vi "Check for DAQ Device.vi"(11 "Physical Channel":tag="Dev1/ai0") -> (0 "error out":errorcluster, 3 "Found?":bool)   [LabVIEW 2011]
doc: "Checks for the specified DAQ device.\n\n\nVersion 1.0 - 02/13/2013\n\nPhaeron, Inc.\nwww.phaeron.com\ninfo@phaeron.com"
uses:
  <vilib>/DAQmx/create/channels.llb/DAQmx Create Channel (AI-Voltage-Basic).vi
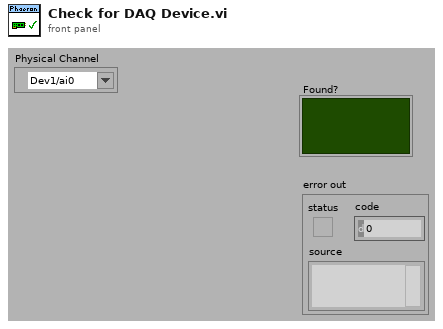
[diagram p1: front panel]
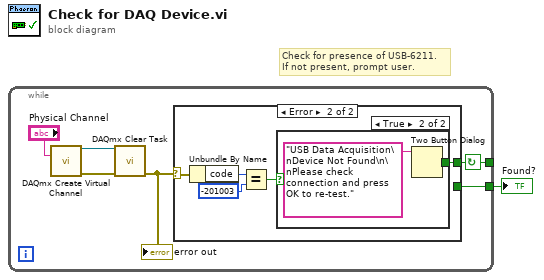
[diagram p0: block diagram]
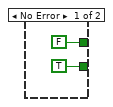
[diagram p2: hidden frame]
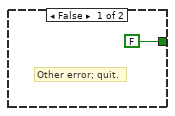
[diagram p3: hidden frame]
diagram:
  # "Check for presence of USB-6211.\nIf not present, prompt user."
  n1 = while {
    tunnel: [w3] -> _
    tunnel: [w2] -> w1
    stop <- w3 continue-if-true
    n2 = call-poly <vilib>:"DAQmx Create Virtual Channel.vi"("physical channels"="Physical Channel") -> ("task out"=w6:refnum<k21>, "error out"=w5:errorcluster)  [unwired: 13 in]
    n3 = call <vilib>:"DAQmx Clear Task.vi"("task in"=w6, "error in"=w5) -> ("error out"=w4:errorcluster)  [unwired: 13 in]
    "error out" <- w4
    n4 = case shown="Error" w4 {
      selector: w4 -> [_ w13]
      tunnel: [FALSE ("T button?") w14] -> w3
      tunnel: [TRUE ("T button?") _] -> w2
      frame No Error {
      }
      frame Error {
        n5 = Unbundle By Name(w13) -> ("code"=w12:i32)
        n6 = Equal?(x=w12, y=-201003) -> (x = y?=w10:bool)
        n7 = case shown="True" w10 {
          tunnel: [FALSE ("T button?") w16] -> w14
          frame False {
            # "Other error; quit."
          }
          frame True {
            n8 = Two Button Dialog(message="USB Data Acquisition\nDevice Not Found\n\nPlease check connection and press OK to re-test.") -> (T button?=w16:bool)  [unwired: 2 in]
          }
        }
      }
    }
  }
  "Found?" <- w1
